vi "WindSpeed.vi"() -> ()   [LabVIEW 2012]
panel:
  out "Wind Speed":dbl
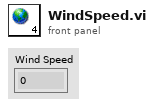
[diagram p1: front panel]
diagram:
